vi "Logging Stopped.vi"(8 "error in (no error)":errorcluster, 10 "Context in":refnum<data-value>, 11 "State in":refnum<class "State.lvclass">) -> (0 "error out":errorcluster, 2 "Context out":refnum<data-value>, 3 "State out":refnum<class "State.lvclass">)   [LabVIEW 2024, in "State.lvlib" / "State.lvclass"]
uses:
  State.lvclass
  State.lvclass/State.ctl
  Context/Context/Context.lvclass
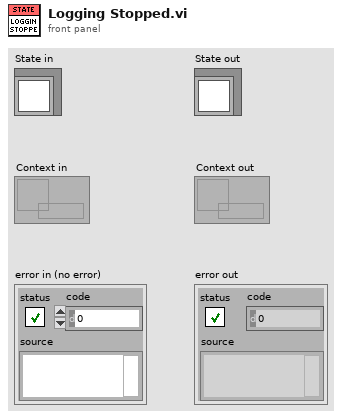
[diagram p1: front panel]
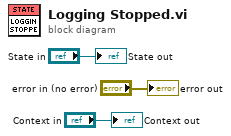
[diagram p0: block diagram]
diagram:
  "error out" <- "error in (no error)"
  "State out" <- "State in"
  "Context out" <- "Context in"
